vi "Remove from Container.vi"(8 "error in (no error)":errorcluster, 11 "GUI View Actor in":refnum<class "GUI View Actor.lvclass">) -> (0 "error out":errorcluster, 3 "GUI View Actor out":refnum<class "GUI View Actor.lvclass">)   [LabVIEW 2023, in "GUI Views.lvlib" / "GUI View Actor.lvclass"]
uses:
  GUI View Actor.lvclass
  GUI View Actor.lvclass/GUI View Actor.ctl
  <vilib>/ActorFramework/Message Enqueuer/Message Enqueuer.lvclass
  View Actor/View Actor.lvclass/View Actor.ctl
  View Actor/properties/Read Name.vi
  properties/Read Managed by Container.vi
  <vilib>/ActorFramework/Message Enqueuer/Equals Not A Refnum.vi
  GUI Container Actor Messages/Remove View Msg/Remove View Msg.lvclass
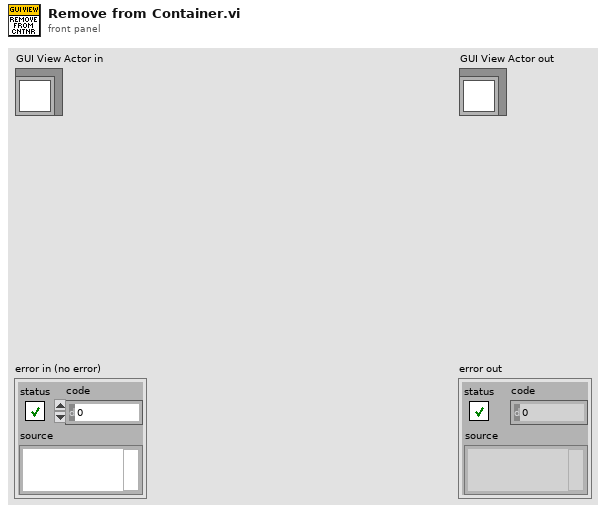
[diagram p1: front panel]
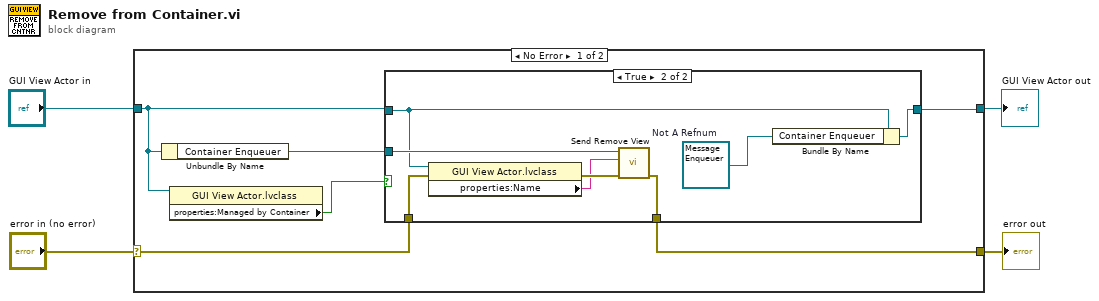
[diagram p0: block diagram]
diagram:
  n1 = case shown="No Error" "error in (no error)" {
    selector: "error in (no error)" -> [w8 w22]
    tunnel: [w7 w22] -> w3
    tunnel: [w9 w21] -> w1
    tunnel: "GUI View Actor in" -> [w6 w21]
    frame No Error {
      n2 = Unbundle By Name(w6) -> ("Container Enqueuer"=w10:refnum<class "Message Enqueuer.lvclass">)
      n3 = property class="GUI View Actor.lvclass"(reference=w6) -> ("properties:Managed by Container"=w5:bool)  [unwired: 1 in, 2 out]
      n4 = case shown="True" w5 {
        tunnel: w10 -> [_ w20]
        tunnel: w6 -> [w12 w15]
        tunnel: [w12 w19] -> w9
        tunnel: w8 -> [w11 w17]
        tunnel: [w11 w13] -> w7
        frame False {
        }
        frame True {
          w18 = refnum<class "Message Enqueuer.lvclass"> refnum  # Not A Refnum
          n5 = property class="GUI View Actor.lvclass"(reference=w15, error in=w17) -> (error out=w16:errorcluster, "properties:Name"=w14:string)  [unwired: 1 out]
          n6 = call "Send Remove View.vi"("error in (no error)"=w16, "View"=w14, "Message Enqueuer in"=w20) -> ("error out"=w13:errorcluster)  [unwired: 7 in, 1 out]
          n7 = Bundle By Name(cluster=w15, "Container Enqueuer"=w18) -> (w19:refnum<class "GUI View Actor.lvclass">)
        }
      }
    }
    frame Error {
    }
  }
  "error out" <- w3
  "GUI View Actor out" <- w1
